vi "Factory.vi"(0 "KObject in":refnum<class "KObject.lvclass">, 7 "Variant":variant, 9 "Prefix":string, 11 "error in (no error)":errorcluster) -> (4 "KObject out":refnum<class "KObject.lvclass">, 8 "Type":string, 15 "error out":errorcluster)   [LabVIEW 2020, in "KObject.lvclass"]
uses:
  KObject.lvclass
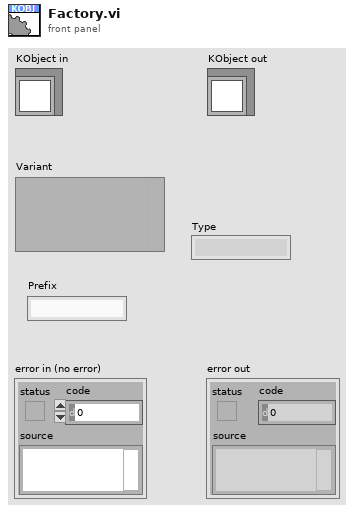
[diagram p1: front panel]
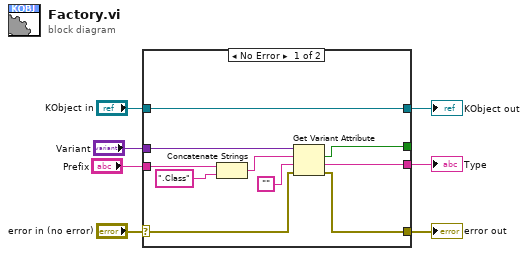
[diagram p0: block diagram]
diagram:
  n1 = case shown="No Error" "error in (no error)" {
    selector: "error in (no error)" -> [w10 w19]
    tunnel: [w9 w19] -> w6
    tunnel: [w13 w18] -> w4
    tunnel: "KObject in" -> [w13 w18]
    tunnel: "Prefix" -> [w17 _]
    tunnel: "Variant" -> [w15 _]
    tunnel: [w11 _] -> w1
    tunnel: [w8 _] -> _
    frame No Error {
      n2 = Concatenate Strings(w17, ".Class" ("string")) -> (w14:string)
      n3 = Get Variant Attribute(Variant=w15, name=w14, default value (empty Variant)="", error in=w10) -> (found=w8:bool, value=w11:string, error out=w9:errorcluster)  [unwired: 1 out]
    }
    frame Error {
    }
  }
  "error out" <- w6
  "KObject out" <- w4
  "Type" <- w1
